vi "Execute Script.vi"(0 "scripts manager in":refnum<class "scripts manager.lvclass">, 11 "error in (no error)":errorcluster) -> (4 "scripts manager out":refnum<class "scripts manager.lvclass">, 15 "error out":errorcluster)   [LabVIEW 2019, in "LSL.lvlib" / "scripts manager.lvclass"]
uses:
  scripts manager.lvclass
  scripts manager.lvclass/scripts manager.ctl
  output terminal/Base/Output Terminal.lvclass
  functions/functionsbase/functionbase.lvclass
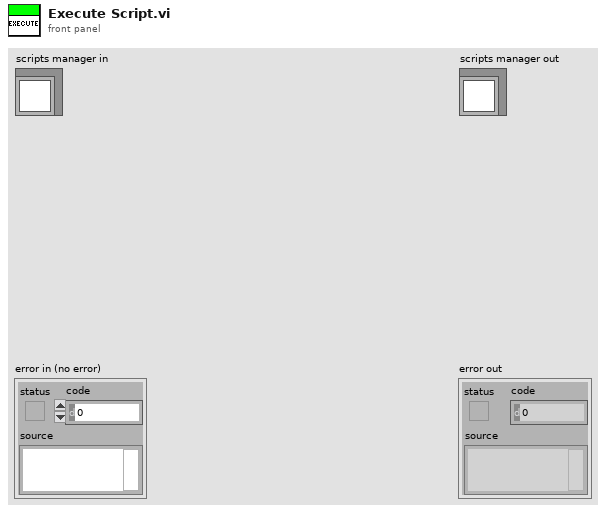
[diagram p1: front panel]
types:
  T1 = typedef "Function Indent Combo.ctl" = cluster{"Parent":refnum<class "functionbase.lvclass">, "Child":refnum<class "functionbase.lvclass">[]}
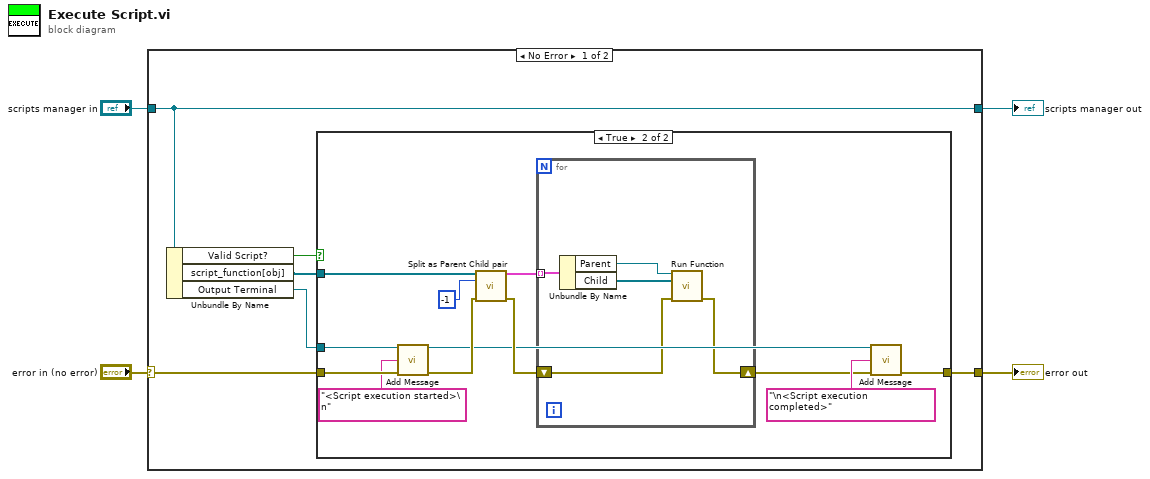
[diagram p0: block diagram]
diagram:
  n1 = case shown="No Error" "error in (no error)" {
    selector: "error in (no error)" -> [w8 w30]
    tunnel: [w7 w30] -> w3
    tunnel: [w10 w29] -> w1
    tunnel: "scripts manager in" -> [w10 w29]
    frame No Error {
      n2 = Unbundle By Name(w10) -> ("Valid Script?"=w6:bool, "script_function[obj]"=w9:refnum<class "functionbase.lvclass">[], "Output Terminal"=w5:refnum<class "Output Terminal.lvclass">)
      n3 = case shown="True" w6 {
        tunnel: w9 -> [_ w23]
        tunnel: w8 -> [w11 w19]
        tunnel: [w11 w12] -> w7
        tunnel: w5 -> [_ w17]
        frame False {
        }
        frame True {
          n4 = call-dynamic "Add Message.vi"("Output Terminal in"=w17, "Message"="<Script execution started>\n", "error in (no error)"=w19) -> ("Output Terminal out"=w14:refnum<class "Output Terminal.lvclass">, "error out"=w18:errorcluster)  [unwired: 11 in]
          n5 = call "Split as Parent Child pair.vi"("Functions"=w23, "Parent Indent"=i64 -1, "error in (no error)"=w18) -> ("Parent Child Combo"=w21:T1[], "error out"=w20:errorcluster)  [unwired: 11 in]
          n6 = for {
            shift-right: [w27] -> w13
            shift-left: w20 -> [w28]
            tunnel: w21 -> [w26] mode=indexing
            n7 = Unbundle By Name(w26) -> ("Parent"=w25:refnum<class "functionbase.lvclass">, "Child"=w24:refnum<class "functionbase.lvclass">[])
            n8 = call-dynamic "Run Function.vi"("functionbase in"=w25, "Sub Functions"=w24, "error in (no error)"=w28) -> ("error out"=w27:errorcluster)  [unwired: 10 in, 2 out]
          }
          n9 = call-dynamic "Add Message.vi"("Output Terminal in"=w14, "Message"="\n<Script execution completed>", "error in (no error)"=w13) -> ("error out"=w12:errorcluster)  [unwired: 11 in, 1 out]
        }
      }
    }
    frame Error {
    }
  }
  "error out" <- w3
  "scripts manager out" <- w1
